vi "Update Record.vi"(8 "error in":errorcluster, 11 "Chronometer in":refnum<class "Chronometer.lvclass">) -> (0 "error out":errorcluster, 3 "Chronometer out":refnum<class "Chronometer.lvclass">)   [LabVIEW 2023, in "Chronometer.lvlib" / "Chronometer.lvclass"]
uses:
  Chronometer.lvclass
  Chronometer.lvclass/Chronometer.ctl
  builds/Tools/Config.lvlibp/Config.lvclass
  C:/Users/Public/Documents/Development/builds/Tools/Config.lvlibp/Config.lvclass
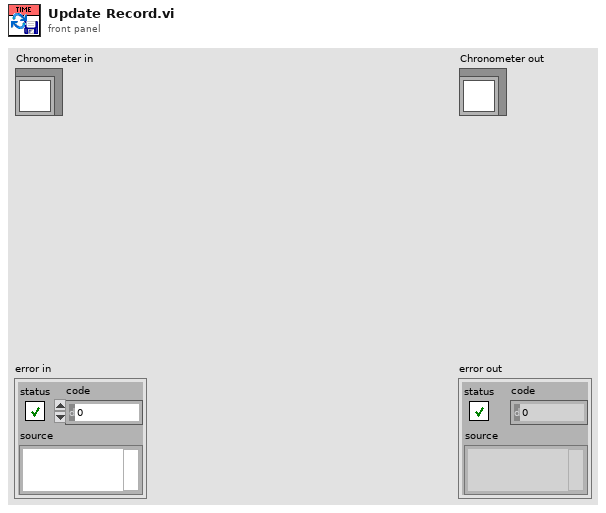
[diagram p1: front panel]
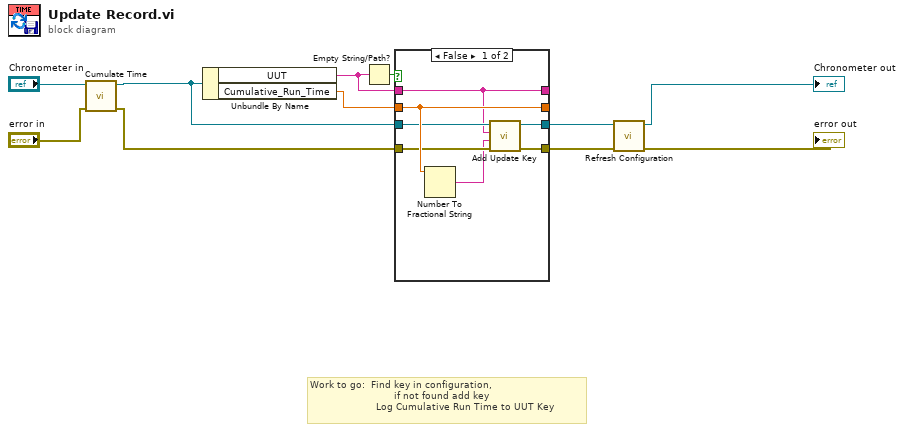
[diagram p0: block diagram]
diagram:
  # "Work to go:  Find key in configuration, \n                            if not found add key\n                      Log Cumulative Run Time to UUT Key"
  n1 = call "Cumulate Time.vi"("error in"="error in", "Chronometer in"="Chronometer in") -> ("error out"=w9:errorcluster, "Chronometer out"=w5:refnum<class "Chronometer.lvclass">)  [unwired: 8 in]
  n2 = Unbundle By Name(w5) -> ("UUT"=w7:string, "Cumulative_Run_Time"=w6:dbl)
  n3 = Empty String/Path?(string/path=w7) -> (empty?=w8:bool)
  n4 = case shown="False" w8 {
    tunnel: w9 -> [w15 w22]
    tunnel: [w14 w22] -> w4
    tunnel: w6 -> [w18 w20]
    tunnel: w7 -> [w12 w21]
    tunnel: [w12 w21] -> _
    tunnel: [w18 w20] -> _
    tunnel: w5 -> [w17 w19]
    tunnel: [w16 w19] -> w3
    frame False {
      n5 = Number To Fractional String(number=w18) -> (F-format string=w13:string)  [unwired: 3 in]
      n6 = call "Add Update Key.vi"("error in"=w15, "Value"=w13, "Key"=w12, "Config in"=w17) -> ("error out"=w14:errorcluster, "Config out"=w16:refnum<class "Chronometer.lvclass">)  [unwired: 6 in]
    }
    frame True {
    }
  }
  n7 = call "Refresh Configuration.vi"("error in"=w4, "Config in"=w3) -> ("error out"=→"error out":errorcluster, "Config out"=→"Chronometer out":refnum<class "Chronometer.lvclass">)  [unwired: 8 in]
